vi "SubVI_CRC_CRCandData.vi"(8 "Error In":errorcluster, 10 "CRC in":u32) -> (0 "Error Out":errorcluster, 1 "CRC out(str)":string, 2 "CRC out":u32)   [LabVIEW 2019]
doc: "Данная VI предназначена для конвертирования пакетов int в string."
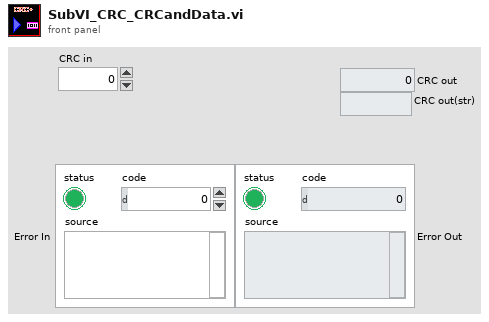
[diagram p1: front panel]
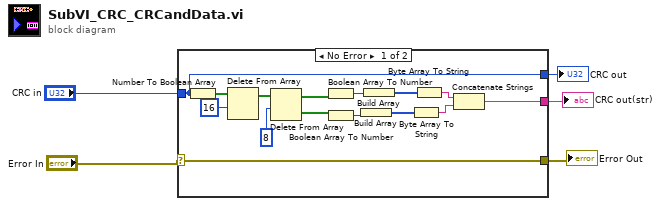
[diagram p0: block diagram]
diagram:
  n1 = case shown="No Error" "Error In" {
    selector: "Error In" -> [w7 w22]
    tunnel: [w20 _] -> w5
    tunnel: "CRC in" -> [w6 w21]
    tunnel: [w7 w22] -> w2
    tunnel: [w6 w21] -> w1
    frame No Error {
      n2 = Number To Boolean Array(number=w6) -> (Boolean array=w15:bool[])
      n3 = Delete From Array(array=w15, length=16) -> (array with subset deleted=w16:bool[])  [unwired: 1 in, 1 out]
      n4 = Delete From Array(array=w16, length=8) -> (deleted portion=w10:bool[], array with subset deleted=w8:bool[])  [unwired: 1 in]
      n5 = Boolean Array To Number(Boolean array=w8) -> (number=w12:u32)
      n6 = Boolean Array To Number(Boolean array=w10) -> (number=w14:u32)
      n7 = Build Array(w14) -> (w13:u32[])
      n8 = Build Array(w12) -> (w11:u32[])
      n9 = Byte Array To String(unsigned byte array=w13) -> (string=w19:string)
      n10 = Byte Array To String(unsigned byte array=w11) -> (string=w18:string)
      n11 = Concatenate Strings(w18, w19) -> (w20:string)
    }
    frame Error {
    }
  }
  "CRC out(str)" <- w5
  "Error Out" <- w2
  "CRC out" <- w1
